vi "TCP Connection Manager.vi"(8 "error in":errorcluster, 9 "method":T4, 10 "index":i32, 11 "connection in":T3) -> (0 "error out":errorcluster, 1 "number of connections":i32, 2 "all connections":T1[](array[typedef]), 3 "connection out":T1)   [LabVIEW 2014]
doc: "This VI maintains the list of host connections."
uses:
  Method.ctl
  Connection.ctl
  <vilib>/NI/STM/SubVIs/MetaDataElement.ctl
  <vilib>/NI/STM/TCP/TCP Connection Info.ctl
  <vilib>/Intelligent Energy/WebSockets API/WebSockets/WebSockets.lvlib
  <vilib>/NI/STM/NI STM.lvlib
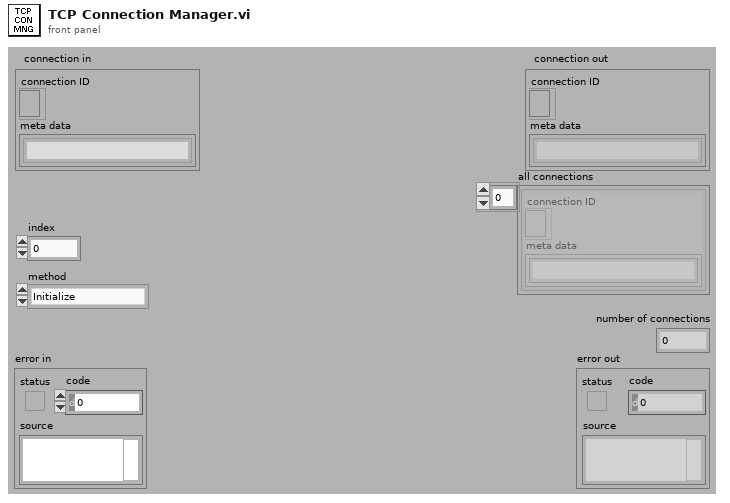
[diagram p1: front panel]
types:
  T1 = typedef "NI STM.lvlib/TCP Connection Info.ctl" = cluster{"connection ID":refnum<k5>, "meta data":T2[]}
  T2 = typedef "NI STM.lvlib/MetaDataElement.ctl" = string
  T3 = typedef "Connection.ctl" = cluster{"connection ID":refnum<k5>, "meta data":T2[]}
  T4 = typedef "Method.ctl" = enum16{"Initialize", "Add Connection", "Set Properties", "Get Connection(s)", "Remove Connection", "Remove All Connections", "Get Connection Count"}
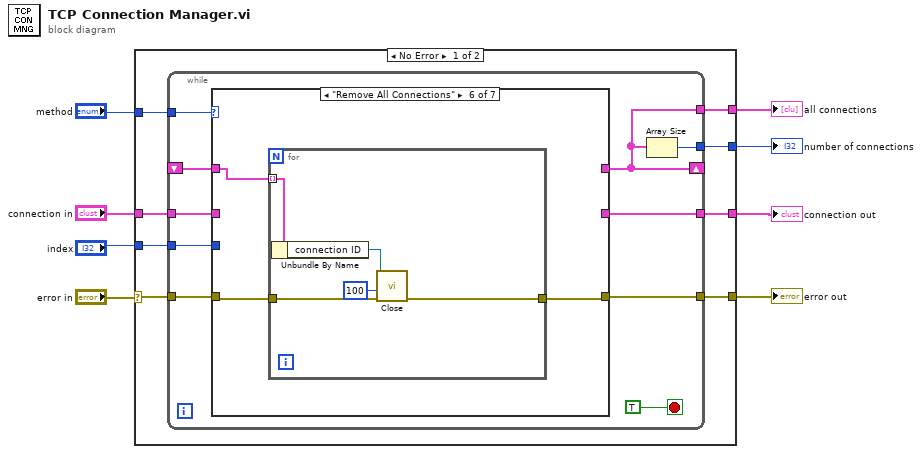
[diagram p0: block diagram]
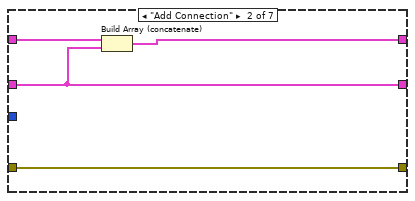
[diagram p3: hidden frame]
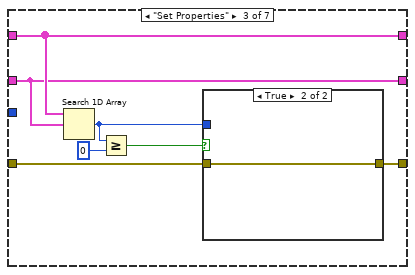
[diagram p4: hidden frame]
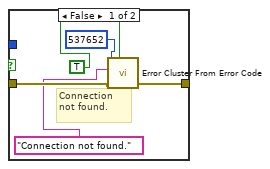
[diagram p5: hidden frame]
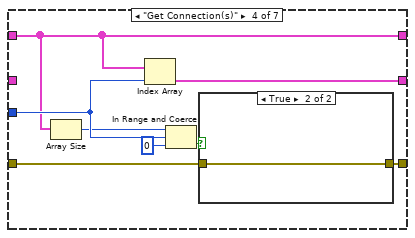
[diagram p6: hidden frame]
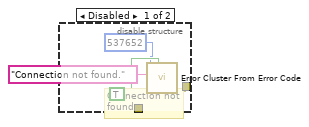
[diagram p8: hidden frame]
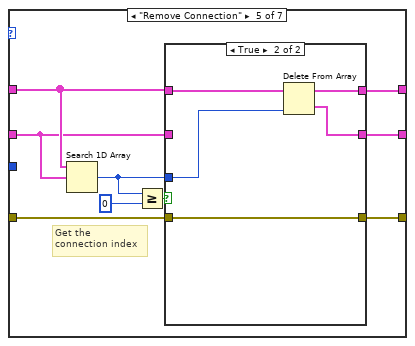
[diagram p9: hidden frame]
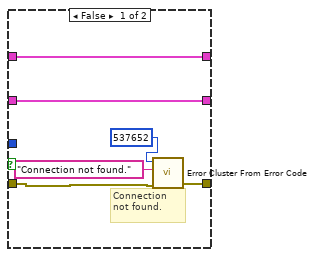
[diagram p10: hidden frame]
diagram:
  n1 = case shown="No Error" "error in" {
    selector: "error in" -> [w16 w94]
    tunnel: [w15 w94] -> w7
    tunnel: "index" -> [w14 _]
    tunnel: "method" -> [w13 _]
    tunnel: "connection in" -> [w12 w93]
    tunnel: [w11 _] -> w3
    tunnel: [w10 _] -> w2
    tunnel: [w9 w93] -> w1
    frame No Error {
      n2 = while {
        shift-right: [w18] -> _
        shift-left: _ -> [w25]
        tunnel: w16 -> [w24]
        tunnel: [w23] -> w15
        tunnel: w14 -> [w22]
        tunnel: w13 -> [w21]
        tunnel: w12 -> [w20]
        tunnel: [w19] -> w11
        tunnel: [w18] -> w10
        tunnel: [w17] -> w9
        stop <- TRUE stop-if-true
        n3 = case shown="\"Remove All Connections\"" w21 {
          tunnel: w25 -> [_ w31 w37 w50 w70 w82 w92]
          tunnel: w20 -> [_ w29 w36 _ w62 _ w91]
          tunnel: [_ w30 w37 w50 w66 _ w92] -> w18
          tunnel: [_ w29 w36 w52 w65 _ w91] -> w17
          tunnel: [w27 w28 w33 w45 w64 w83 w90] -> w23
          tunnel: w24 -> [w27 w28 w34 w48 w63 w84 w90]
          tunnel: w22 -> [_ _ _ w51 _ _ _]
          frame "Initialize" {
          }
          frame "Add Connection" {
            n4 = Build Array (concatenate)(w31, w29) -> (w30:T3[])
          }
          frame "Set Properties" {
            n5 = Search 1D Array(1D array=w37, element=w36) -> (index of element=w32:i32)  [unwired: 1 out]
            n6 = Greater Or Equal?(x=w32, y=0) -> (x >= y?=w35:bool)
            n7 = case shown="True" w35 {
              tunnel: w34 -> [w42 w44]
              tunnel: [w43 w44] -> w33
              tunnel: w32 -> [_ _]
              frame False {
                # "Connection not found."
                n8 = call <vilib>:"Error Cluster From Error Code.vi"("show call chain? (False)"=TRUE ("status (T)"), "error in (no error)"=w42, "error message (\"\")"="Connection not found.", "error code (0)"=537652 ("code")) -> ("error out"=w43:errorcluster)  [unwired: 5 in]
              }
              frame True {
              }
            }
          }
          frame "Get Connection(s)" {
            n9 = Array Size(array=w50) -> (size(s)=w49:i32)
            n10 = Index Array(array=w50, index=w51) -> (element=w52:T3)
            n11 = In Range and Coerce(upper limit=w49, x=w51, lower limit=0) -> (In Range?=w47:bool)  [unwired: 1 out]
            n12 = case shown="True" w47 {
              tunnel: w48 -> [w54 w61]
              tunnel: [w53 w61] -> w45
              frame False {
                n13 = disable-structure shown="Enabled" {
                  disable-tunnel: w54 -> [w58 w60]
                  disable-tunnel: [w57 w60] -> w53
                  frame Disabled {
                    # "Connection not found."
                    n14 = call <vilib>:"Error Cluster From Error Code.vi"("show call chain? (False)"=TRUE ("status (T)"), "error in (no error)"=w58, "error message (\"\")"="Connection not found." ("error message (\"\")"), "error code (0)"=537652 ("code")) -> ("error out"=w57:errorcluster)  [unwired: 5 in]
                  }
                  frame Enabled {
                  }
                }
              }
              frame True {
              }
            }
          }
          frame "Remove Connection" {
            # "Get the \nconnection index"
            n15 = Search 1D Array(1D array=w70, element=w62) -> (index of element=w69:i32)  [unwired: 1 out]
            n16 = Greater Or Equal?(x=w69, y=0) -> (x >= y?=w67:bool)
            n17 = case shown="True" w67 {
              tunnel: w70 -> [w76 w80]
              tunnel: w69 -> [_ w79]
              tunnel: [w76 w81] -> w66
              tunnel: [w75 w78] -> w65
              tunnel: [w73 w77] -> w64
              tunnel: w63 -> [w72 w77]
              tunnel: w62 -> [w75 _]
              frame False {
                # "Connection not found."
                n18 = call <vilib>:"Error Cluster From Error Code.vi"("error in (no error)"=w72, "error message (\"\")"="Connection not found." ("error message (\"\")"), "error code (0)"=537652 ("code")) -> ("error out"=w73:errorcluster)  [unwired: 6 in]
              }
              frame True {
                n19 = Delete From Array(array=w80, index=w79) -> (deleted portion=w78:T3, array with subset deleted=w81:T3[])  [unwired: 1 in]
              }
            }
          }
          frame "Remove All Connections" {
            n20 = for {
              tunnel: w84 -> [w88]
              tunnel: [w87] -> w83
              tunnel: w82 -> [w86] mode=indexing
              n21 = Unbundle By Name(w86) -> ("connection ID"=w85:refnum<k5>)
              n22 = call <vilib>:"Close.vi"("error in (no error)"=w88, "timeout ms (5000)"=100, "WebSocket Connection in"=w85) -> ("error out"=w87:errorcluster)  [unwired: 7 in, 1 out]
            }
          }
          frame "Get Connection Count" {
          }
        }
        n23 = Array Size(array=w18) -> (size(s)=w19:i32)
      }
    }
    frame Error {
    }
  }
  "error out" <- w7
  "number of connections" <- w3
  "all connections" <- w2
  "connection out" <- w1
